vi "Create Deadband vi.vi"(2 "Input Deadband":dbl, 3 "Input":dbl, 4 "Output Upper Limit":dbl format="%#_13g") -> (0 "Output":dbl)   [LabVIEW 2015]
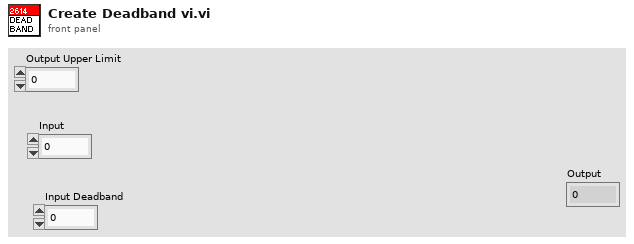
[diagram p1: front panel]
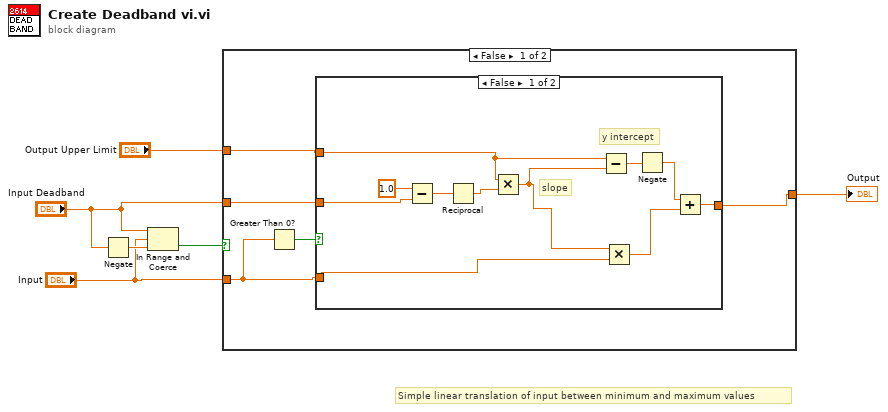
[diagram p0: block diagram]
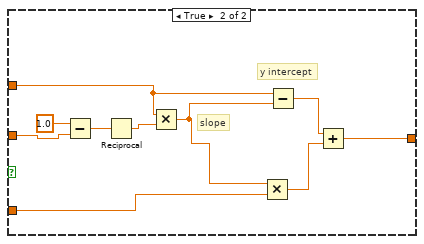
[diagram p2: hidden frame]
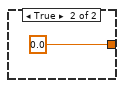
[diagram p3: hidden frame]
diagram:
  # "Simple linear translation of input between minimum and maximum values"
  n1 = Negate(x="Input Deadband") -> (-x=w6:dbl)
  n2 = In Range and Coerce(upper limit="Input Deadband", x="Input", lower limit=w6) -> (In Range?=w3:bool)  [unwired: 1 out]
  n3 = case shown="False" w3 {
    tunnel: "Input Deadband" -> [w10 _]
    tunnel: "Input" -> [w7 _]
    tunnel: [w9 0.0 ("Output")] -> w2
    tunnel: "Output Upper Limit" -> [w11 _]
    frame False {
      n4 = Greater Than 0?(x=w7) -> (x > 0?=w8:bool)
      n5 = case shown="False" w8 {
        tunnel: w11 -> [w17 w29]
        tunnel: w10 -> [w18 w28]
        tunnel: w7 -> [w16 w27]
        tunnel: [w15 w24] -> w9
        frame False {
          # "y intercept"
          # "slope"
          n6 = Subtract(x=1.0, y=w18) -> (x-y=w20:dbl)
          n7 = Reciprocal(x=w20) -> (1/x=w21:dbl)
          n8 = Multiply(x=w17, y=w21) -> (x*y=w12:dbl)
          n9 = Subtract(x=w17, y=w12) -> (x-y=w14:dbl)
          n10 = Multiply(x=w12, y=w16) -> (x*y=w22:dbl)
          n11 = Negate(x=w14) -> (-x=w13:dbl)
          n12 = Add(x=w13, y=w22) -> (x+y=w15:dbl)
        }
        frame True {
          # "y intercept"
          # "slope"
          n13 = Subtract(x=1.0, y=w28) -> (x-y=w31:dbl)
          n14 = Reciprocal(x=w31) -> (1/x=w30:dbl)
          n15 = Multiply(x=w29, y=w30) -> (x*y=w23:dbl)
          n16 = Multiply(x=w23, y=w27) -> (x*y=w26:dbl)
          n17 = Subtract(x=w29, y=w23) -> (x-y=w25:dbl)
          n18 = Add(x=w25, y=w26) -> (x+y=w24:dbl)
        }
      }
    }
    frame True {
    }
  }
  "Output" <- w2
